vi "Image Upload.vi"(0 "Sift Client in":refnum<class "Sift Client.lvclass">, 1 "Filepath":string, 2 "Entity ID":string, 3 "Entity Type":T2, 4 "Description":string, 5 "error in (no error)":errorcluster, 7 "Width":i32, 9 "Height":i32) -> (14 "Sift Client out":refnum<class "Sift Client.lvclass">, 19 "error out":errorcluster)   [LabVIEW 2024, in "Sift Client.lvlib" / "Sift Client.lvclass"]
doc: "Uploads an image file pointed to by Filepath and attaches it to the provided Entity ID. Optionally include the image width and height for optimal viewing experience in the Sift application."
uses:
  Sift Client.lvclass
  Private/Typedefs/Messages/File Attachment Upload Request.ctl
  Types/Entity Type.ctl
  Private/Typedefs/Messages/Video Metadata.ctl
  Private/Typedefs/Messages/Image Metadata.ctl
  Private/Typedefs/Messages/Metadata Type.ctl
  Private/Typedefs/Messages/JSON Request.ctl
  Sift Client.lvclass/Sift Client.ctl
  Sift Client.lvlib
  <vilib>/addons/_JKI.lib/Serialization/JSON/JKI JSON Serialization.lvlib
panel:
  in  "image_metadata":T1
  in  "JSON Request":T3
  in  "File Attachment Upload Request":T4
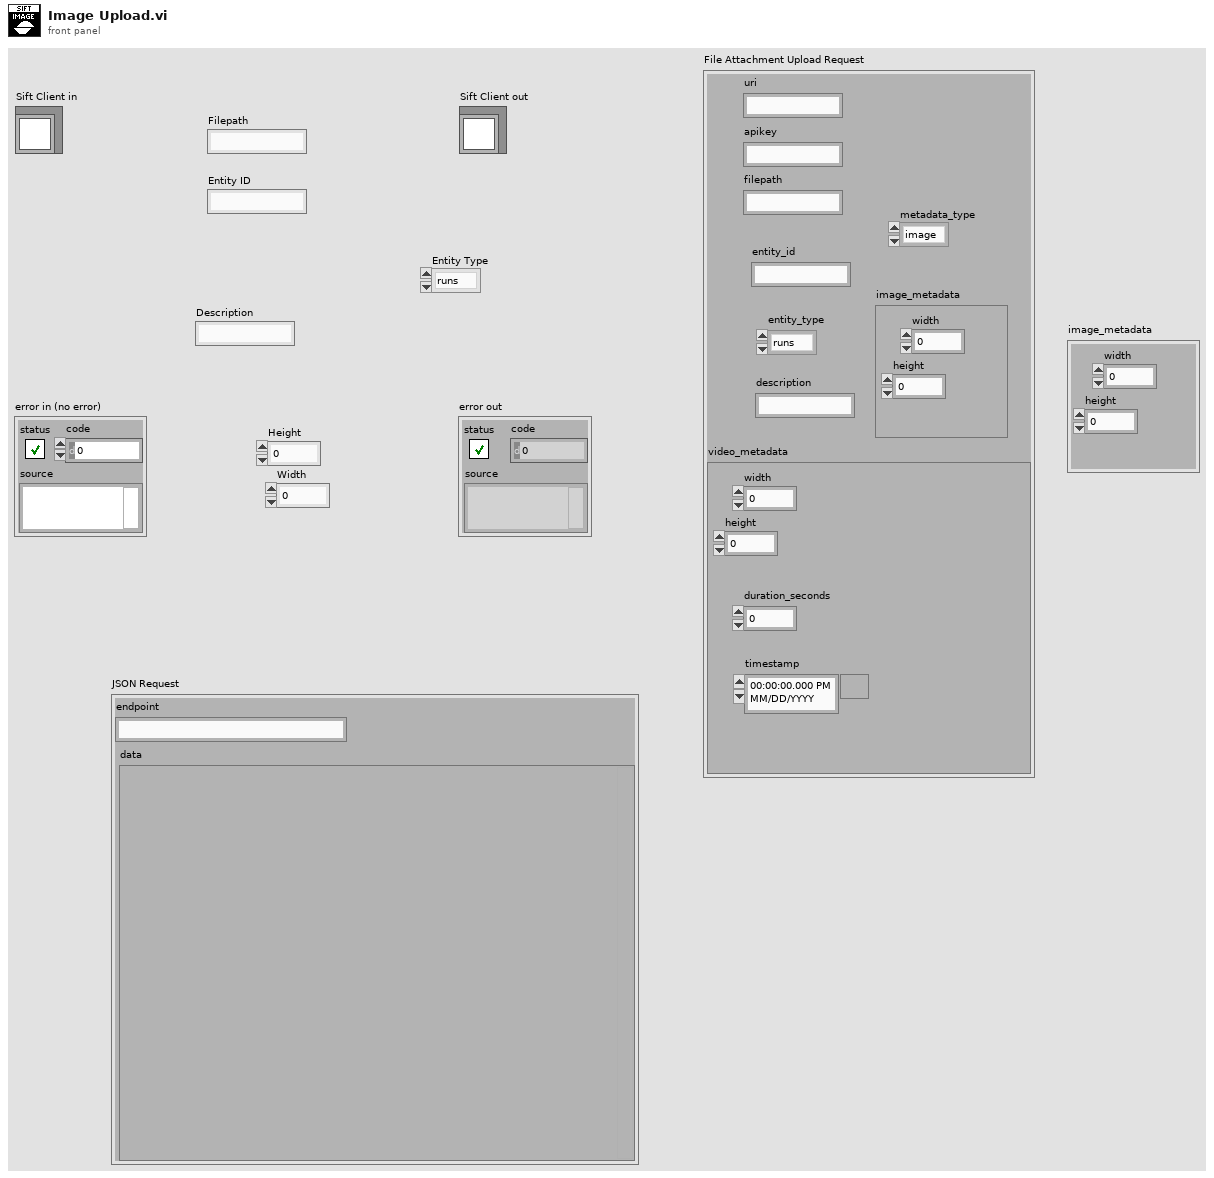
[diagram p1: front panel]
types:
  T1 = typedef "Sift Client.lvlib/Image Metadata.ctl" = cluster{"height":i32, "width":i32}
  T2 = typedef "Sift Client.lvlib/Entity Type.ctl" = enum16{"runs", "annotations", "annotation_logs"}
  T3 = typedef "Sift Client.lvlib/JSON Request.ctl" = cluster{"endpoint":string, "data":variant}
  T4 = typedef "Sift Client.lvlib/File Attachment Upload Request.ctl" = cluster{"uri":string, "apikey":string, "filepath":string, "entity_id":string, "description":string, "entity_type":T2, "video_metadata":T5, "image_metadata":T1, "metadata_type":T6}
  T5 = typedef "Sift Client.lvlib/Video Metadata.ctl" = cluster{"duration_seconds":dbl, "timestamp":timestamp, "height":i32, "width":i32}
  T6 = typedef "Sift Client.lvlib/Metadata Type.ctl" = enum16{"image", "video"}
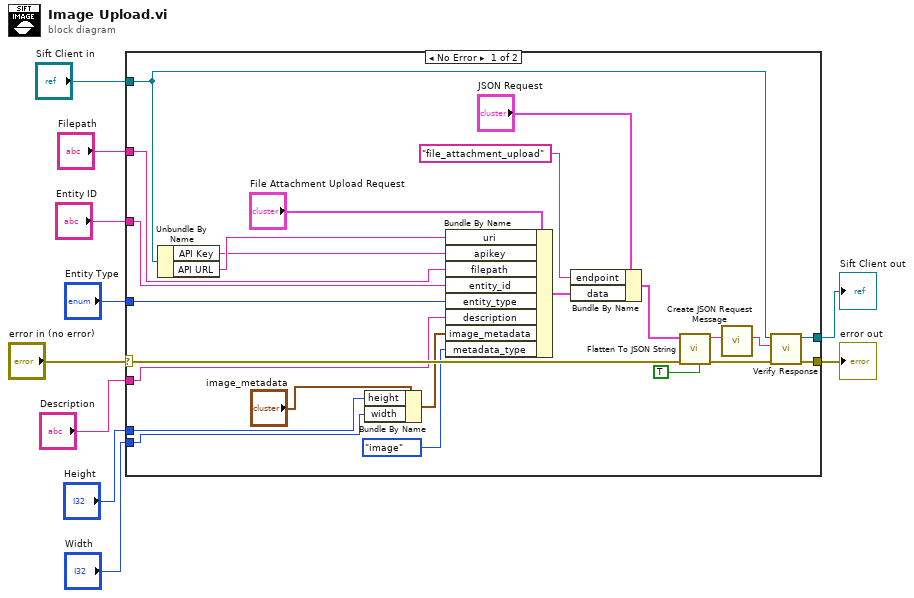
[diagram p0: block diagram]
diagram:
  n1 = case shown="No Error" "error in (no error)" {
    selector: "error in (no error)" -> [w26 w36]
    tunnel: [w25 w36] -> w9
    tunnel: [w24 w35] -> w7
    tunnel: "Sift Client in" -> [w13 w35]
    tunnel: "Entity Type" -> [w21 _]
    tunnel: "Entity ID" -> [w20 _]
    tunnel: "Filepath" -> [w19 _]
    tunnel: "Description" -> [w18 _]
    tunnel: "Height" -> [w17 _]
    tunnel: "Width" -> [w16 _]
    frame No Error {
      n2 = Unbundle By Name(w13) -> ("API Key"=w22:string, "API URL"=w23:string)
      n3 = Bundle By Name(cluster="image_metadata", "height"=w17, "width"=w16) -> (w15:T1)
      n4 = Bundle By Name(cluster="File Attachment Upload Request", "uri"=w23, "apikey"=w22, "filepath"=w19, "entity_id"=w20, "entity_type"=w21, "description"=w18, "image_metadata"=w15, "metadata_type"=Metadata_Type."image") -> (w32:T4)
      n5 = Bundle By Name(cluster="JSON Request", "endpoint"="file_attachment_upload", "data"=w32) -> (w27:T3)
      n6 = call <vilib>:"Flatten To JSON String.vi"("Enums As String (F)"=TRUE, "error in"=w26, "Variant"=w27) -> ("error out"=w28:errorcluster, "JSON String"=w30:string)  [unwired: 7 in]
      n7 = call "Create JSON Request Message.vi"("Data"=w30) -> ("Message"=w29:string)  [unwired: 10 in]
      n8 = call-dynamic "Verify Response.vi"("error in (no error)"=w28, "Message"=w29, "Sift Client in"=w13) -> ("error out"=w25:errorcluster, "Sift Client out"=w24:refnum<class "Sift Client.lvclass">)  [unwired: 6 in, 1 out]
    }
    frame Error {
    }
  }
  "error out" <- w9
  "Sift Client out" <- w7
